vi "Control.vi"(8 "error in (no error)":errorcluster, 11 "Teleop_Lift in":refnum<class "Teleop_Lift.lvclass">) -> (0 "error out":errorcluster, 2 "Setpoint Reached?":bool, 3 "Teleop_Lift out":refnum<class "Teleop_Lift.lvclass">)   [LabVIEW 2018, in "Teleop_Lift.lvclass"]
uses:
  Teleop_Lift.lvclass
  <vilib>/Rock Robotics/WPI/ThirdParty/Phoenix-LabVIEW/Motor Controller/Controls/CTRE_Phoenix_MotorControl_ControlMode.ctl
  Teleop_Lift.lvclass/Teleop_Lift.ctl
  513cbc10-7326-459d-9587-05ba751338aa.vi
  <vilib>/Rock Robotics/WPI/ThirdParty/Phoenix-LabVIEW/Motor Controller/Get/CTRE_Phoenix_MotorController_GetQuadratureData.vi
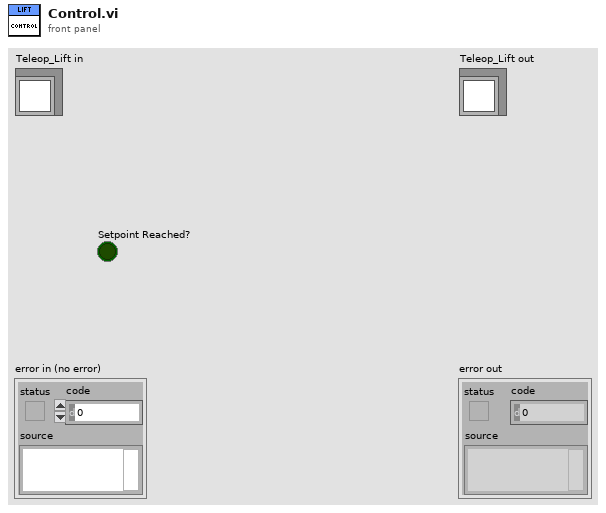
[diagram p1: front panel]
types:
  T1 = typedef "CTRE_Phoenix_MotorControl_ControlMode.ctl" = u16
  T2 = typedef "WPI_MotorControlDeviceRef.ctl" = cluster{"DeviceStatus":errorcluster, "Type":T3, "PWM":cluster{"PWM Channel":T4, "DeadBand":T5}, "CAN":cluster{"Device Number":u8, "SetOutput VI Ref":variant, "GetOutput VI Ref":variant, "Enable VI Ref":variant, "Disable VI Ref":variant, "Data":variant}, "Invert":bool, "DIO PWM":cluster{"PWM \"Enable\" Channel":T4, "DIOChannel":T6, "PWM Rate":dbl}}
  T3 = typedef "WPI_MotorControlType.ctl" = enum16{"PWM", "CAN", "DIO PWM"}
  T4 = typedef "FPGA_DIOPWMChannel.ctl" = enum8{"PWM 0", "PWM 1", "PWM 2", "PWM 3", "PWM 4", "PWM 5", "PWM 6", "PWM 7", "PWM 8", "PWM 9", "PWM MXP 0", "PWM MXP 1", "PWM MXP 2", "PWM MXP 3", "PWM MXP 4", "PWM MXP 5", "PWM MXP 6", "PWM MXP 7", "PWM MXP 8", "PWM MXP 9", "Invalid"}
  T5 = typedef "WPI_PWMDeadband.ctl" = cluster{"Name":string, "maxPositivePwm":i32, "minPositivePwm":i32, "centerPwm":i32, "maxNegativePwm":i32, "minNegativePwm":i32, "angularRange":u16}
  T6 = typedef "FPGA_DIOChannel.ctl" = enum8{"DIO 0", "DIO 1", "DIO 2", "DIO 3", "DIO 4", "DIO 5", "DIO 6", "DIO 7", "DIO 8", "DIO 9", "DIO MXP 0", "DIO MXP 1", "DIO MXP 2", "DIO MXP 3", "DIO MXP 4", "DIO MXP 5", "DIO MXP 6", "DIO MXP 7", "DIO MXP 8", "DIO MXP 9", "DIO MXP 10", "DIO MXP 11", "DIO MXP 12", "DIO MXP 13", "DIO MXP 14", "DIO MXP 15", "SPI Port CS1", "SPI Port CS2", "SPI Port CS3", "SPI Port MISO", "SPI Port MOSI", "Invalid"}
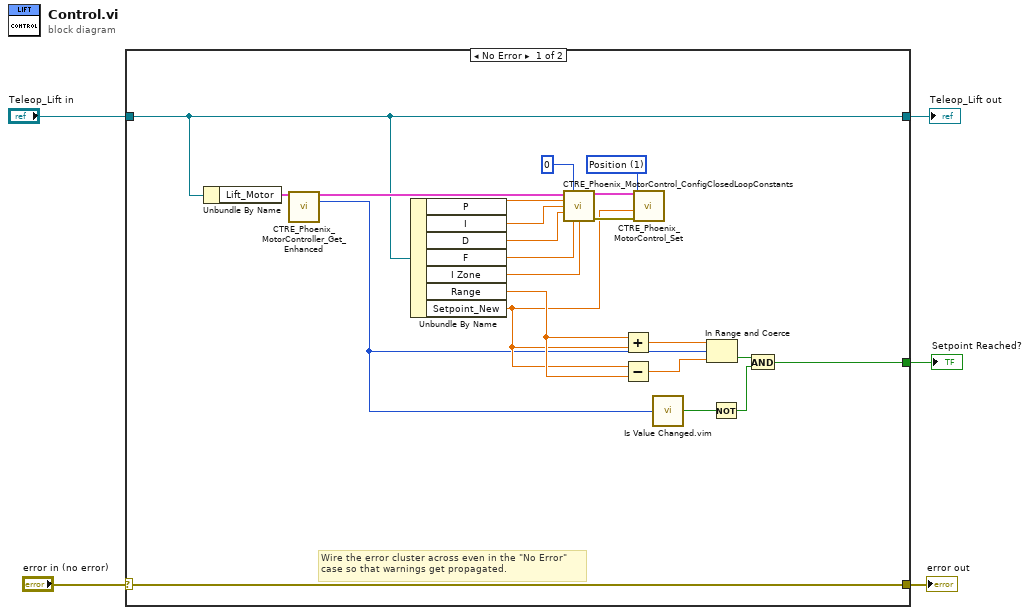
[diagram p0: block diagram]
diagram:
  n1 = case shown="No Error" "error in (no error)" {
    selector: "error in (no error)" -> [w27 w29]
    tunnel: [w27 w29] -> w4
    tunnel: [w24 w28] -> w2
    tunnel: "Teleop_Lift in" -> [w24 w28]
    tunnel: [w6 _] -> w1
    frame No Error {
      w15 = T1 1 items=["PercentOutput"=0, "Position"=1, "Velocity"=2, "Current"=3, "Follower"=5, "MotionProfile"=6, "MotionMagic"=7, "MotionProfileArc"=10, "Disabled"=15] ("Control Mode")
      # "Wire the error cluster across even in the \"No Error\"\ncase so that warnings get propagated."
      n2 = Unbundle By Name(w24) -> ("Lift_Motor"=w26:T2)
      n3 = call-poly <vilib>:"CTRE_Phoenix_MotorController_Get_Enhanced.vi"("PhoenixMotorControlDevRef"=w26) -> ("PhoenixMotorControlDevRef"=w25:T2, "Quadrature Position"=w7:i32)  [unwired: 11 in, 2 out]
      n4 = Unbundle By Name(w24) -> ("P"=w23:dbl, "I"=w22:dbl, "D"=w21:dbl, "F"=w20:dbl, "I Zone"=w19:dbl, "Range"=w9:dbl, "Setpoint_New"=w8:dbl)
      n5 = call <vilib>:"CTRE_Phoenix_MotorControl_ConfigClosedLoopConstants.vi"("PhoenixMotorControlDevRef"=w25, "slotIdx"=0, "P"=w23, "I"=w22, "D"=w21, "F"=w20, "I Zone"=w19) -> ("PhoenixMotorControlDevRef"=w16:T2, "error out"=w17:errorcluster)  [unwired: 7 in]
      n6 = Add(x=w9, y=w8) -> (x+y=w13:dbl)
      n7 = Subtract(x=w8, y=w9) -> (x-y=w14:dbl)
      n8 = call <vilib>:"CTRE_Phoenix_MotorControl_Set.vi"("error in (no error)"=w17, "Output"=w8, "Control Mode"=w15, "PhoenixMotorControlDevRef"=w16) -> ()  [unwired: 6 in, 2 out]
      n9 = call "Is Value Changed.vim"("value"=w7) -> ("changed or first call?"=w10:bool)
      n10 = In Range and Coerce(upper limit=w13, x=w7, lower limit=w14) -> (In Range?=w12:bool)  [unwired: 1 out]
      n11 = Not(x=w10) -> (.not. x?=w11:bool)
      n12 = And(x=w12, y=w11) -> (x .and. y?=w6:bool)
    }
    frame Error {
    }
  }
  "error out" <- w4
  "Teleop_Lift out" <- w2
  "Setpoint Reached?" <- w1
